vi "Show.vi"(8 "error in":errorcluster, 11 "Flex Subpanel in":refnum<class "Flex UI Subpanel.lvclass">) -> (0 "error out":errorcluster, 3 "Flex Subpanel out":refnum<class "Flex UI Subpanel.lvclass">)   [LabVIEW 2016, in "Flex UI Subpanel.lvclass"]
doc: "Shows the UI."
uses:
  Flex UI Subpanel.lvclass
  Flex UI Subpanel.lvclass/Flex UI Subpanel.ctl
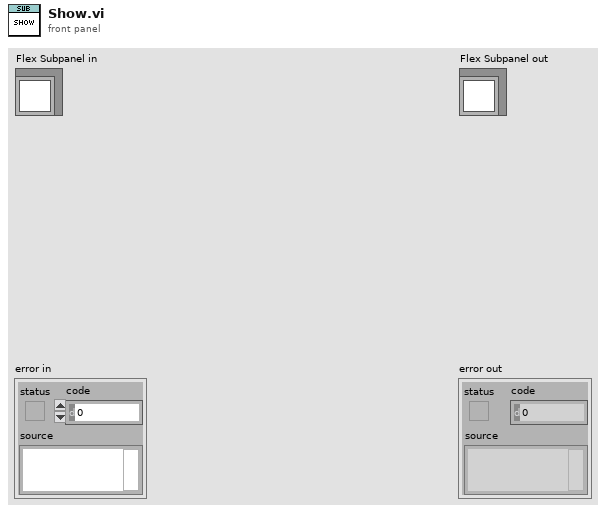
[diagram p1: front panel]
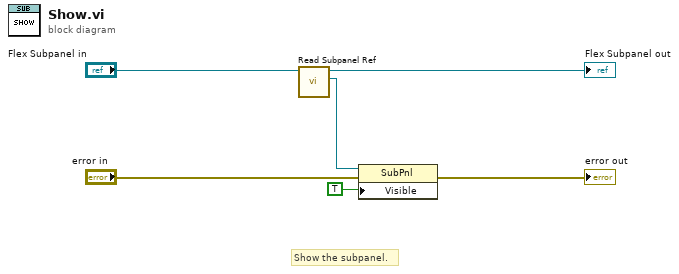
[diagram p0: block diagram]
diagram:
  # "Show the subpanel."
  n1 = call "Read Subpanel Ref.vi"("Flex Subpanel in"="Flex Subpanel in") -> ("Subpanel Ref"=w5:refnum<vi>, "Flex Subpanel out"=→"Flex Subpanel out":refnum<class "Flex UI Subpanel.lvclass">)  [unwired: 9 in]
  n2 = property class="SubPnl"(reference=w5, error in="error in", "Visible"=TRUE) -> (error out=→"error out":errorcluster)  [unwired: 1 out]
